vi "LAC pharse Msg (SubVI).vi"(2 "result":string) -> (0 "array out":string[](array[string]), 1 "ERR?":bool)   [LabVIEW 8.6]
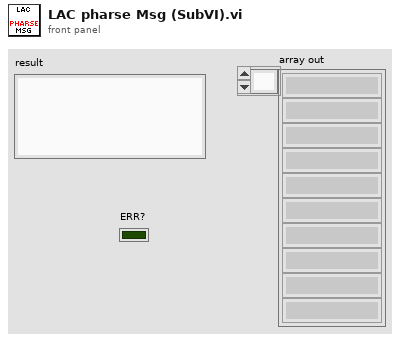
[diagram p1: front panel]
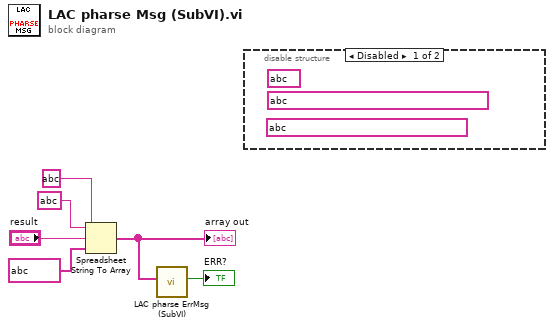
[diagram p0: block diagram]
diagram:
  n1 = Spreadsheet String To Array(delimiter (Tab)=string ?, format string=string ?, spreadsheet string="result", array type (2D Dbl)=string[] ?) -> (array=w2:string[])
  "array out" <- w2
  n2 = call "LAC pharse ErrMsg (SubVI).vi"("Response"=w2) -> ("ERR?"=→"ERR?":bool)  [unwired: 8 in, 2 out]
  n3 = disable-structure shown="Disabled" {
    frame #0 {
      (unwired) string ?
      (unwired) string ?
      (unwired) string ?
    }
    frame #1 {
    }
  }
